vi "SetDigRej.vi"(8 "错误输入（无错误）":errorcluster, 11 "检波模式索引值":u8) -> (0 "错误输出":errorcluster)   [LabVIEW 2014]
uses:
  X86Dll/ZXUTConfigMgr.dll
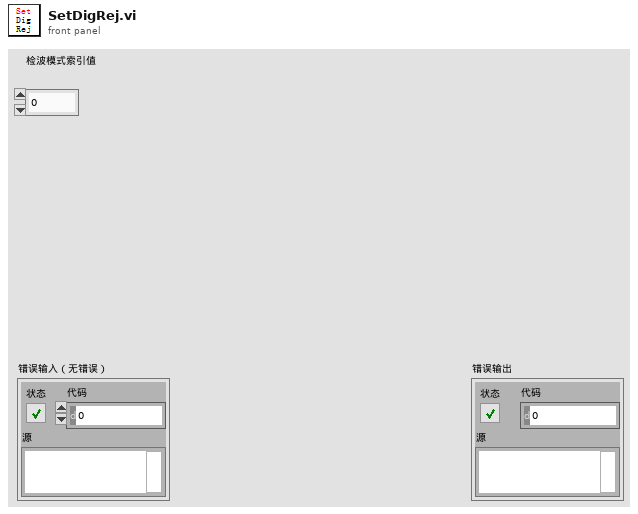
[diagram p1: front panel]
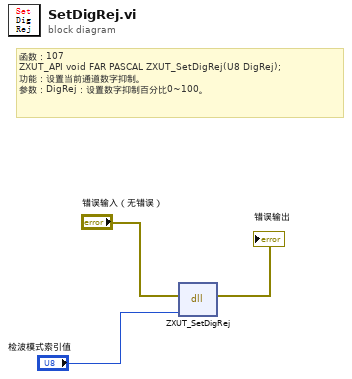
[diagram p0: block diagram]
diagram:
  # "函数：107\nZXUT_API void\tFAR PASCAL ZXUT_SetDigRej(U8 DigRej);\n功能：设置当前通道数字抑制。\n参数：DigRej：设置数字抑制百分比0~100。"
  n1 = dll-call lib="D:/Software/Utrasonic on-line monitoring/X86Dll/ZXUTConfigMgr.dll" fn="ZXUT_SetDigRej"(error in="错误输入（无错误）", "DigRej"="检波模式索引值") -> (error out=→"错误输出":errorcluster)  [unwired: 4 in, 1 out]
